vi "Main.vi"() -> ()   [LabVIEW 2016]
panel:
  in  "Changelog":string="LASER MARKING\nWabco & T&M Solutions\nMaciej Szupienko (maciej.szupienko@wabco-auto.com)\nKrzysztof Krypczyk (krzysztof.krypczyk@averna.com)\n------------------------------------------------------------------------------\nTODO:\n- More plates than 2 in one order\n- Results - record the reason of NOK\n- Prod.Take - check why Sucker isn't turned on again before checking presence\n- consider removing tunning and tune only for golden samples\n- sometimes missing data matrix coordinates overlay (probably scanner problem)\n- add laser error commands (after updating laser firmware to v1.5 by videojet)\n------------------------------------------------------------------------------\n\nv1.0.9 (MSZ 2018-05-24)\n- add bank A/B-3 for scania client plates\n- correct image and overlay display\n\nv1.0.8 (MSZ 2018-03-26)\n- add summary popup gui after every plate order in double order\n\nv1.0.7 (MSZ 2018-03-23)\n- while opening door move ProdLift and ProdArm to base positions (to prevent the plate to fall to OK container when arm is holding the plates)\n- correct v1.0.6\n- try 5 times to unload the table then popup pause err msg\n- for double order do not change to the client plate when stopped (this also solved problem with continuoing the order when stopped)\n- when using global counter fix restarting the order when stopped\n- correct laser loop shutdown\n- use Proda time for log events/errors\n- add pause/resume/door open/door close log events\n- remove sql_error.txt at shutdown\n- correct ProdArm move\n\nv1.0.6 (MSZ 2018-03-21)\n- while unloading when plate is holded by the arm check also sensor in the slot (if there is another plate, move holing plate and the one in the slot to the NOK)\n\nv1.0.5 (MSZ 2018-03-19)\n- correct method of approving serial numbers after table rotation\n\nv1.0.4 (MSZ 2018-03-09)\n- correct Q5 move (arm move to work position)\n\nv1.0.3 (MSZ 2018-03-09)\n- correct DMC config validation\n\nv1.0.2 (MSZ 2017-11-22)\n- remove empty jobs from laser jobs list (while selecting empty job errow as returned)\n- extend laser connection timeout from 3 to 15 sec\n- change the default loaded laser job at app startup\n\nv1.0.1 (MSZ 2017-10-30)\n- stable release\n- option to ignore WabcoNo formatting (for special orders)\n\nv0.49 (MSZ 2017-10-24)\n- update global counter after each plate and not after order completed to prevent dupliactes if order is stopped or aborted\n\nv0.48.4 (MSZ 2017-09-18)\n- write the variants file with backup if changed\n- archive old variants files\n- partOK confirm bugfix\n\nv0.48.3 (MSZ 2017-09-04)\n- choose bank for scanner (A/B-1 as 1,2 and A/B-2 as 3,4)\n\nv0.48.2 (MSZ 2017-09-04)\n- update serial number list to be saved to file while station is in error or stopped (to prevent duplicate plates while resuming)\n\nv0.48.1 (MSZ 2017-08-23)\n- accept signs 'O', 'P', 'R' in wabco number (for Provia plates)\n\nv0.47 (MSZ 2017-08-16)\n- correct rotating table - when error do not rotate software buffer - to avoid duplicates\n- correct translation file\n\nv0.46 (MSZ 2017-07-27)\n- correct unloading phase (simplify the code and checking for the product)\n- while unloading & loading wait for averaging the sensor data in the buffer\n- add durations of each slot to the tdms file\n- show serial number when ignored\n- do not ignore the samples in slot 2 & 3 (can be done only in 1 and 4)\n- when \"Check DMC\" is off then scan only once\n- correct statistics gui\n\nv0.45.1 (MSZ 2017-07-20)\n- minor final status correction (sometimes it was still NOK after OK)\n\nv0.45 (MSZ 2017-07-20)\n- v0.44 did not solve duplicates\n- add 350ms delay after OK Drop before next presence sensor read out (digital outputs are using buffered avaraging and need time to update the value0 - sample was dropped to OK, then sensor read out by mistake that the sample is stiill there and overrride its status to NOK\n- additional prevent in serial buffer (to count OK/NOK only for the serial numbers with or without Verification to prevent overriding the status of OK sample)\n\nv0.44 (MSZ 2017-07-19)\n- minor changes to prevent from duplicates\n\nv0.43 (MSZ 2017-06-14)\n- if plate is not unloaded due to the error then mark the plate as OK or NOK (operator should manually put the plate into correct container)\n- check for DMC when Serial is defined in laser template\n- restore back timeout of table rotation to 5 sec (pre-home to 500ms)\n\nv0.42 (MSZ 2017-06-14)\n- when test starts set Rotations=0 and CodeReady=False\n- auto archive variant ini file every 1 day\n- bugfix while rotating the table and status clean (many duplicates)\n- extend timeout of table rotation from o5 to 7,5 sec (pre-home to 750ms)\n\nv0.41 (MSZ 2017-06-13)\n- correct unloading process and plate status control while error at unloading (when error occured at unloading do not update the status of the plate)\n- while rotating the table if the previous unloaded plate is still pending then it is marked as FAILED\n\nv0.40 (MSZ 2017-06-05)\n- add images folder to archiver\n- set archiver period to 90 days for images and 365 days for tdms files (configurable in Config.ini file)\n- add error when free HD disk space is below 1GB\n\nv0.39 (MSZ 2017-05-29)\n- replace R to 0 in variant number after scanning\n\nv0.38 (MSZ 2017-05-12)\n- if there is an error while droping the plate down to the OK container then marked this plate as passed always to avoid duplicates\n- retry if the code was not read properly or threshold was too low\n- add short err code beside the code about the failure\n- after scanning the code write the result of scanning and not the expected code\n\nv0.37 (MSZ 2017-05-06)\n- correct Drop action (extend the period of blowing and reduce delay elsewhere)\n- time range in statistics gui\n- show only plates with any results in statistics gui\n- change errors into pause warnings while unloading (test needed)\n- add pause source info (A,B, A/B)\n\nv0.36 (MSZ 2017-04-28)\n- add process status to log file\n- do not move file if order is stopped or aborted\n\nv0.35 (MSZ 2017-04-26)\n- add table and graph in statistics GUI\n\nv0.34 (MSZ 2017-04-25)\n- add first statistics based on files\n\nv0.33 (MSZ 2017-04-25)\n- do not show last part done message\n- correct TS of the first plates\n\nv0.32 (MSZ 2017-04-24)\n- connect to process from proda and save results to proda\n- use proda time for results if available\n\nv0.31 (MSZ 2017-04-21)\n- save global counter after process is completed; it helps to restart the the process properly based on prior global counter\n- add part indicator at test step gui\n\nv0.30 (MSZ 2017-04-14)\n- continue with proda export (not finished yet)\n\nv0.29 (MSZ 2017-04-14)\n- connection to proda\n- name of the station\n\nv0.28 (MSZ 2017-04-13)\n- partial order\n- correct the way of counting parts\n\nv0.27 (MSZ 2017-04-12)\n- added wabco icon\n- add OrderQuantity in Order (not programmed yet)\n- tested DMC configurator and DMC printing\n- added StationNo in config.ini to distinguish the stations\n- use common ini files except of the Variants.ini which has number of the station\n- renamed variants into plates and store there only plate images\n- move Variants.ini file to settings folder and delete unused files\n\nv0.26 (MSZ 2017-04-11)\n- upgrade to LV2016\n- replace TMS with Wabco logo\n- remove size of dmc component\n- check component size base on the laser setup (not tested)\n\nv0.25 (MSZ 2017-04-10)\n- added DMC (data matrix code) configurator screen\n- Summary GUI after job done\n- prepare Statistics GUI\n\nv0.24 (MSZ 2017-03-13)\n- clear +1 week option when order is done or new order accepted\n\nv0.23 (MSZ 2017-03-01)\n- if order has serial number do not add it to the range of serial number but print it directly as it is\n- add \"+1 week\" button in the process start gui, then add +1 week to the date in the plate\n\nv0.22 (KrKr 2016-11-04)\n- Prod.DropNOK/OK: increment fail/pass counter only if FinalA/B=false\n- Prod.DropNOK/OK: increment fail/pass counter even if error during dropping\n- Prod.DropNOK/OK: error order reflected in \"Pause status\"\n- Keyence.Main-Scan.Product: logic fixed\n- Sequence.Test.Unload - status propagation fix when Wait On NOK/OK\n\nv0.21 (KK 2016-09-12)\n- Laser marking timeout situation handled\n- Daq.Gui: V7310.File.Write disabled (Laser.ini read-only)\n\nv0.20 (KK 2016-07-05)\n- MainGui: Scanner Panel button in Process Mode to access tuning\n- KeyenceGui: AutoTune button aded to turn automatic tuning on/off (Config.ini)\n- KeyenceGui: Most options disabled when at Operator level\n\nv0.19 (KK 2016-06-23)\n- Unload OK: Check Prod -> Lift Down -> Blow Out -> Check Prod -> Lift Up\n- Unload OK/NOK: 250ms wait after ArmLift Work (before blow out)\n\nv0.18 (KK 2016-06-06)\n- Added Product BlowOut A/B signals to help unload products\n- BlowOut signals activated only at Final product unloading\n- ArmLift goes down before turning underpressure off for NOK & OK\n\nv0.17 (2016-05-20)\n- correct failures limit\n- tunnedB missing while starting new order\n- disable door lock button while container is missing\n- extend class indicator in diagnostics screen\n\nv0.16 (2016-03-30)\n- (MSZ) close the order after it is done - go to order screen automatically\n- (MSZ) narrow the range of scanners\n- (MSZ) added translation file for Poliish\n- (MSZ) if serial number is not scanned put -1 to the control value and give warning; serial number type changed from U32 to I32\n- (MSZ) center client product number in the plate printing\n- (MSZ) laser empty program (000 000 000 0) for testing revolvers\n\nv0.15 (2016-03-23)\n- (MSZ) correct stopping action while being in pause mode\n- (MSZ) correct table rotation function\n\nv0.14 (2016-03-22)\n- (MSZ) add archiver loop\n- (MSZ) remove spaces in order start number and quantity\n- (MSZ) handle nexpected table position in home procedure\n- (MSZ) extend timeout after reaching position before blocking\n\nv0.13 (2016-03-18)\n- (MSZ) change 'NOK container missing' inito 'OK container missing'\n- (MSZ) correct double order counters\n- (MSZ) correct log file\n\nv0.12 (2016-03-16)\n- (MSZ) tune scanner when failed in reading\n- (MSZ) convert some errors into warnings + pause during sequence\n- (MSZ) if only one nest has product for the first time put system in pause\n- (MSZ) correct date\n\nv0.11 (2016-03-09)\n- (MSZ) correct laser SetJob function (remove unnecessary CRLF)\n\nv0.10 (2016-02-25)\n- log clean messages from laser\n\nv0.9 (2016-02-23)\n- execution of double order\n- continue with aborted order\n- laser programs\n\nv0.8 (2016-02-19)\n- offset for laser for station\n- continue file after application restart\n- restart scanner on startup in runtime mode\n- standby laser state (set to 60sec)\n\nv0.7 (2016-02-11)\n- changeover screen and configuration modified\n\nv0.6 (2016-02-11)\n- max failures limit with auto pause when limit is exceeded\n- unlock door button in main screen while in pause\n\nv0.5 (2016-01-28)\n- configure order scanner\n- integrate order scanner with changeover screen\n\nv0.4 (2016-01-21)\n- changed DI/DO order\n- added DI S.C Front Door Secured\n- define slot ID order at startup\n- logger loop\n\nv0.3 (2015-12-21)\n- results screen\n- sequence loop\n- station loop\n\nv0.2 (2015-11-09)\n- converted to LV2015\n- manual screen and VIs\n- keyence scanner loop\n\nv0.1 (2015-11-02)\n- application core" caption="MAKE CURRENT VALUE DEFAULT!!!"
  # ">>>MAIN<<<"
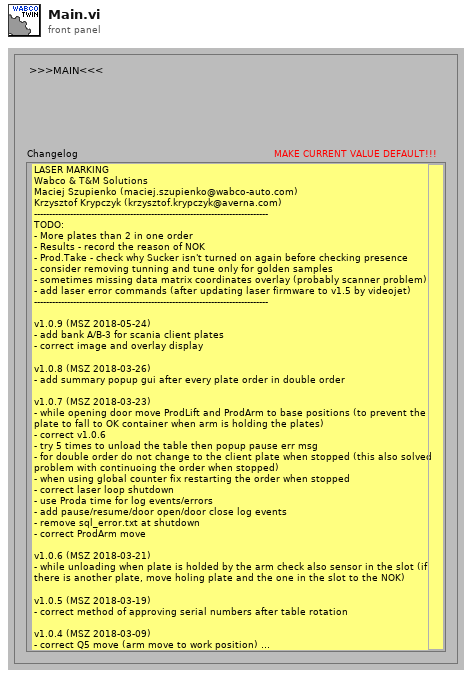
[diagram p1: front panel]
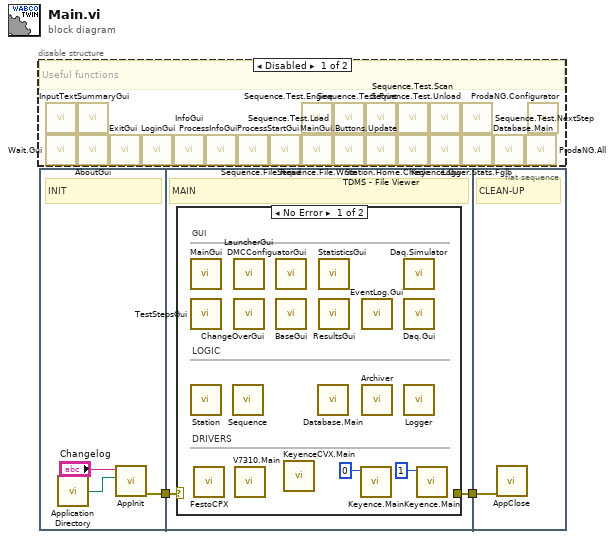
[diagram p0: block diagram]
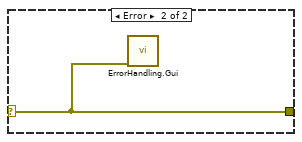
[diagram p3: hidden frame]
diagram:
  n1 = disable-structure shown="Disabled" {
    frame Disabled {
      # "Useful functions"
      n2 = call "InputText.vi"() -> ()  [unwired: 11 in, 1 out]
      n3 = call "Wait.Gui.vi"() -> ()  [unwired: 12 in]
      n4 = call "SummaryGui.vi"() -> ()  [unwired: 12 in]
      n5 = call "AboutGui.vi"() -> ()  [unwired: 12 in]
      n6 = call "ExitGui.vi"() -> ()  [unwired: 10 in, 2 out]
      n7 = call "LoginGui.vi"() -> ()  [unwired: 11 in, 1 out]
      n8 = call "InfoGui.vi"() -> ()  [unwired: 11 in, 1 out]
      n9 = call "ProcessInfoGui.vi"() -> ()  [unwired: 10 in, 2 out]
      n10 = call "ProcessStartGui.vi"() -> ()  [unwired: 10 in, 2 out]
      n11 = call "Sequence.File.Read.vi"() -> ()  [unwired: 10 in, 2 out]
      n12 = call "Sequence.Test.Engine.vi"() -> ()  [unwired: 10 in, 2 out]
      n13 = call "Sequence.File.Write.vi"() -> ()  [unwired: 11 in, 1 out]
      n14 = call "Sequence.Test.Load.vi"() -> ()  [unwired: 10 in, 2 out]
      n15 = call "MainGui.Buttons.Update.vi"() -> ()  [unwired: 11 in, 1 out]
      n16 = call "Sequence.Test.Print.vi"() -> ()  [unwired: 10 in, 2 out]
      n17 = call <vilib>:"TDMS - File Viewer.vi"() -> ()  [unwired: 6 in, 2 out]
      n18 = call "Sequence.Test.Scan.vi"() -> ()  [unwired: 10 in, 2 out]
      n19 = call "Station.Home.Check.vi"() -> ()  [unwired: 7 in, 5 out]
      n20 = call "Sequence.Test.Unload.vi"() -> ()  [unwired: 10 in, 2 out]
      n21 = call "Keyence.Gui.vi"() -> ()  [unwired: 11 in, 1 out]
      n22 = call "Sequence.Test.NextStep.vi"() -> ()  [unwired: 9 in, 3 out]
      n23 = call "Logger.Stats.Fglb.vi"() -> ()  [unwired: 10 in, 2 out]
      n24 = call "Database.Main.vi"() -> ()  [unwired: 1 in]
      n25 = call "ProdaNG.All.vi"() -> ()  [unwired: 12 in]
      n26 = call "ProdaNG.Configurator.vi"() -> ()  [unwired: 12 in]
    }
    frame Enabled {
    }
  }
  n27 = flat-sequence {
    tunnel: [w3] -> w2
    tunnel: w2 -> [w7]
    tunnel: [w6] -> w1
    tunnel: w1 -> [w11]
    frame #0 {
      # "INIT"
      n28 = call <vilib>:"Application Directory.vi"() -> ("Application Directory"=w4:path)
      n29 = call "AppInit.vi"("path"=w4, "Changelog"="Changelog") -> ("error out"=w3:errorcluster)  [unwired: 9 in]
    }
    frame #1 {
      # "MAIN"
      n30 = case shown="No Error" w7 {
        selector: w7 -> [_ w10]
        tunnel: [_ w10] -> w6
        frame No Error {
          # "GUI"
          # "LOGIC"
          # "DRIVERS"
          n31 = call "MainGui.vi"() -> ()  [unwired: 1 in]
          n32 = call "TestStepsGui.vi"() -> ()  [unwired: 12 in]
          n33 = call "Station.vi"() -> ()  [unwired: 12 in]
          n34 = call "FestoCPX.vi"() -> ()  [unwired: 12 in]
          n35 = call "Sequence.vi"() -> ()  [unwired: 12 in]
          n36 = call "LauncherGui.vi"() -> ()  [unwired: 12 in]
          n37 = call "ChangeOverGui.vi"() -> ()  [unwired: 12 in]
          n38 = call "V7310.Main.vi"() -> ()  [unwired: 1 in]
          n39 = call "DMCConfiguatorGui.vi"() -> ()  [unwired: 12 in]
          n40 = call "BaseGui.vi"() -> ()  [unwired: 12 in]
          n41 = call "KeyenceCVX.Main.vi"() -> ()  [unwired: 12 in]
          n42 = call "Database.Main.vi"() -> ()  [unwired: 1 in]
          n43 = call "StatisticsGui.vi"() -> ()  [unwired: 12 in]
          n44 = call "ResultsGui.vi"() -> ()  [unwired: 12 in]
          n45 = call "Keyence.Main.vi"("idx"=0) -> ()  [unwired: 11 in]
          n46 = call "EventLog.Gui.vi"() -> ()  [unwired: 12 in]
          n47 = call "Archiver.vi"() -> ()  [unwired: 12 in]
          n48 = call "Daq.Simulator.vi"() -> ()  [unwired: 12 in]
          n49 = call "Daq.Gui.vi"() -> ()  [unwired: 12 in]
          n50 = call "Logger.vi"() -> ()  [unwired: 12 in]
          n51 = call "Keyence.Main.vi"("idx"=1) -> ()  [unwired: 11 in]
        }
        frame Error {
          n52 = call "ErrorHandling.Gui.vi"("error in (no error)"=w10) -> ()  [unwired: 9 in, 2 out]
        }
      }
    }
    frame #2 {
      # "CLEAN-UP"
      n53 = call "AppClose.vi"("error in (no error)"=w11) -> ()  [unwired: 11 in]
    }
  }
